vi "Get Available Channels.vi"(8 "error in (no error)":errorcluster, 11 "NI DAQ in":refnum<class "NI DAQ.lvclass">) -> (0 "error out":errorcluster, 3 "NI DAQ out":refnum<class "NI DAQ.lvclass">)   [LabVIEW 2015, in "NI DAQ.lvlib" / "NI DAQ.lvclass"]
uses:
  NI DAQ.lvclass
  Sequencer/Sequencer/Daq Channel Info.ctl
  IO Device/IO Device/IO Device.lvclass
  <resource>/objmgr/daqmx.rc
  Sequencer/Sequencer/Sequencer.lvclass
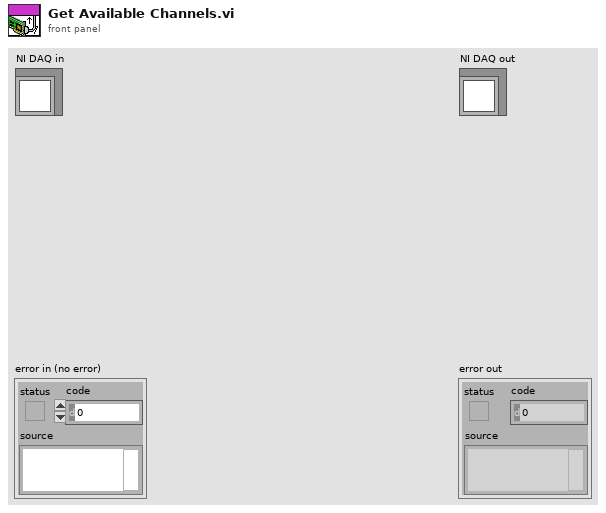
[diagram p1: front panel]
types:
  T1 = typedef "Sequencer.lvlib/Sequencer.lvclass/Daq Channel Info.ctl" = cluster{"DevNames":tag[], "AO.PhysicalChans":tag[][], "DO.Lines":tag[][], "AI.PhysicalChans":tag[][]}
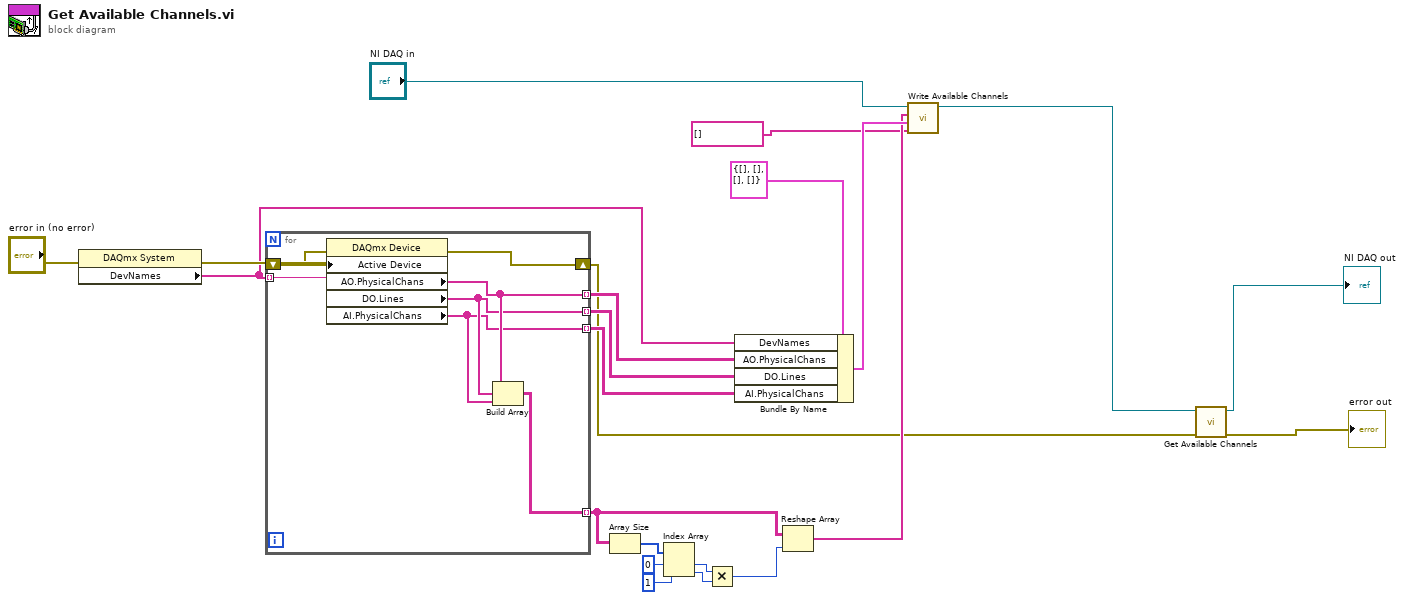
[diagram p0: block diagram]
diagram:
  n1 = property class="DAQmx System"(error in="error in (no error)") -> (error out=w19:errorcluster, "DevNames"=w18:tag[])  [unwired: 1 in, 1 out]
  n2 = for {
    tunnel: w18 -> [w29] mode=indexing
    tunnel: [w26] -> w15 mode=indexing
    tunnel: [w25] -> w16 mode=indexing
    tunnel: [w24] -> w17 mode=indexing
    shift-right: [w27] -> w2
    shift-left: w19 -> [w28]
    tunnel: [w23] -> w9 mode=indexing
    n3 = property class="DAQmx Device"(error in=w28, "Active Device"=w29) -> (error out=w27:errorcluster, "AO.PhysicalChans"=w26:tag[], "DO.Lines"=w25:tag[], "AI.PhysicalChans"=w24:tag[])  [unwired: 1 in, 1 out]
    n4 = Build Array(w26, w25, w24) -> (w23:tag[][])
  }
  n5 = Array Size(array=w9) -> (size(s)=w14:i32[])
  n6 = Index Array(array=w14, index #1=0 ("index"), index #2=1 ("index")) -> (element #1=w11:i32, element #2=w10:i32)
  n7 = Multiply(x=w11, y=w10) -> (x*y=w8:i32)
  n8 = Bundle By Name(cluster=T1 {"DevNames"=[], "AO.PhysicalChans"=[], "DO.Lines"=[], "AI.PhysicalChans"=[]} ("DAQ Channel Info"), "DevNames"=w18, "AO.PhysicalChans"=w15, "DO.Lines"=w16, "AI.PhysicalChans"=w17) -> (w6:T1)
  n9 = Reshape Array(w9, w8) -> (w5:tag[])
  n10 = call "Write Available Channels.vi"("IO Device in"="NI DAQ in", "All Daq Channels"=w5, "DAQ Channel Info"=w6, "Used DAQChannels"=tag[] []) -> ("IO Device out"=w1:refnum<class "NI DAQ.lvclass">)  [unwired: 6 in]
  n11 = call-parent "Get Available Channels.vi"("error in (no error)"=w2, "IO Device in"=w1) -> ("error out"=→"error out":errorcluster, "IO Device out"=→"NI DAQ out":refnum<class "NI DAQ.lvclass">)  [unwired: 8 in]
